vi "Arduino Stepper Motor v1.vi"() -> ()   [LabVIEW 2019, in "LabVIEW Interface for Arduino.lvlib"]
doc: "This example shows how to use the Arduino Stepper Motor API. The fritzing diagram shows use with the EasyStepper 4.3 or 4.4 motor controller."
uses:
  <vilib>/LabVIEW Interface for Arduino/LabVIEW Interface for Arduino.lvlib
  <vilib>/LabVIEW Interface for Arduino/Type Defs/Connection Type.ctl
  <vilib>/LabVIEW Interface for Arduino/Type Defs/Board Type.ctl
  <vilib>/LabVIEW Interface for Arduino/Type Defs/Pin Mode.ctl
panel:
  in  "Motor Enable/Disable":bool
  in  "Stop":bool
  in  "Stepper #":u8=1
  in  "OK Button":bool
  in  "Set Acceleration (0 to disable)":i16
  in  "# of Steps to Move":i16
  in  "Set Speed (Steps per Second)":i16=100
  out "Steps Remaining?":bool
  in  "Dial":i16(knob) scale=0.0..200.0
  in  "error in":errorcluster
  # "Preset Movement"
  # "Interactive Movement"
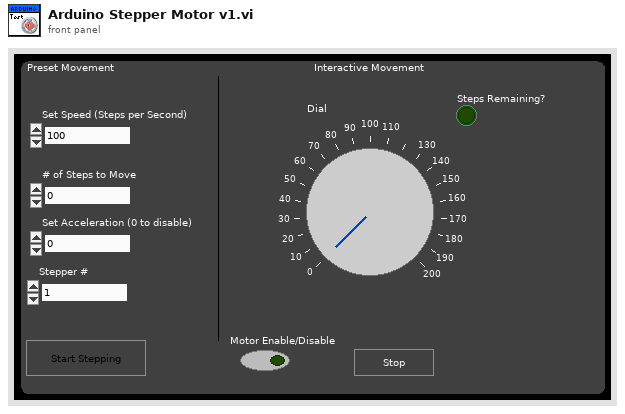
[diagram p1: front panel]
types:
  T1 = typedef "LabVIEW Interface for Arduino.lvlib/Board Type.ctl" = enum16{"Uno", "Dimuelanove w/Atmega 328", "Mega 2560"}
  T2 = typedef "LabVIEW Interface for Arduino.lvlib/Connection Type.ctl" = enum8{"USB / Serial", "XBEE", "BlueSmirf (Bluetooth)"}
  T3 = typedef "LabVIEW Interface for Arduino.lvlib/Arduino Resource.ctl" = cluster{"VISA resource":refnum<visa-resource-name>, "Board Type":T1, "Connection Type":enum8{"USB / Serial"}, "Bytes Per Packet (15)":u8}
  T4 = typedef "LabVIEW Interface for Arduino.lvlib/Pin Mode.ctl" = enum8{"Input", "Output"}
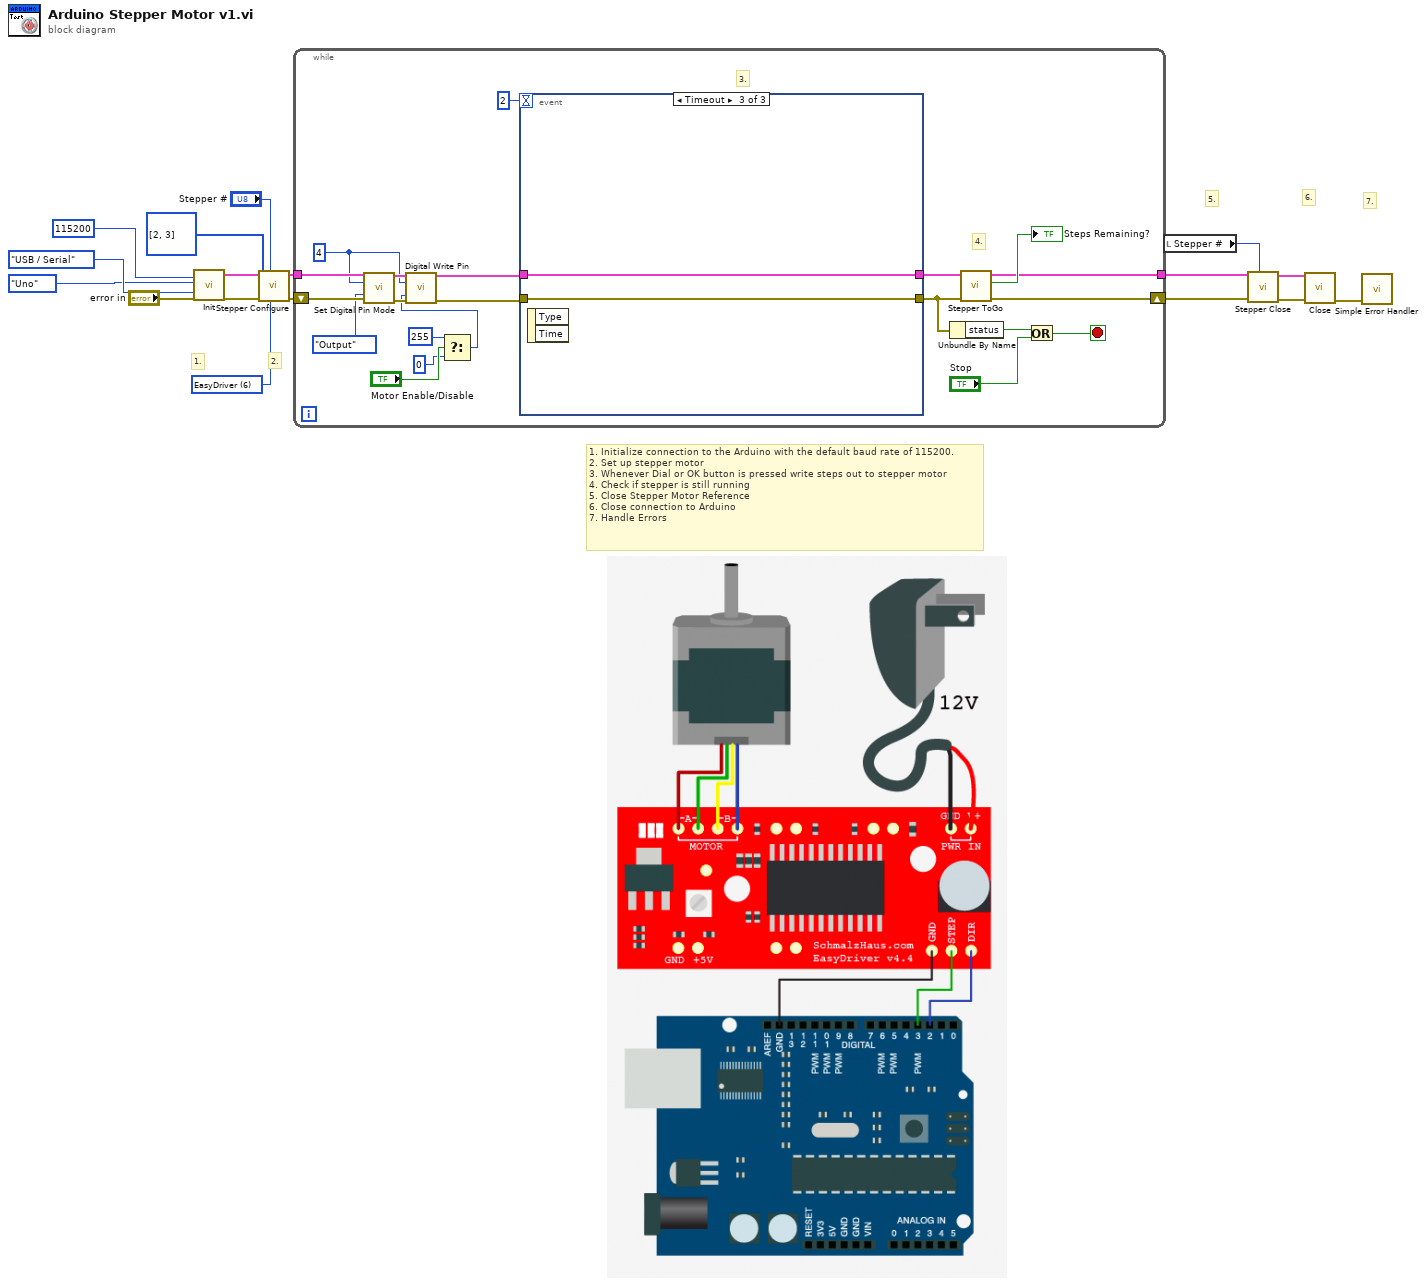
[diagram p0: block diagram]
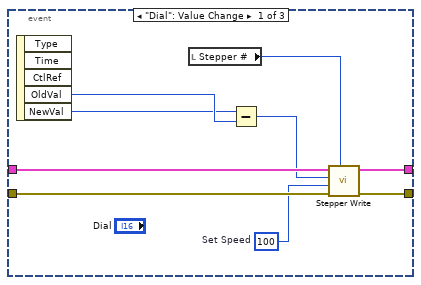
[diagram p2: hidden frame]
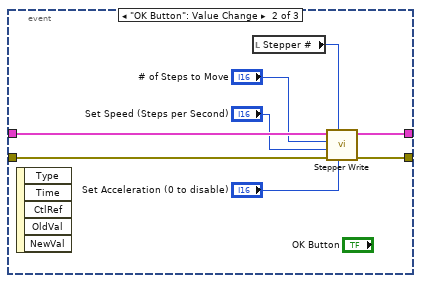
[diagram p3: hidden frame]
diagram:
  w4 = u8 6 items=["2 Wire (Pulse & Direction)"=1, "2 Wire"=2, "4 Wire"=4, "EasyDriver"=6, "AF Motor Shield (Stepper 1 & 2 Only)"=5] ("Control Method")
  # "7."
  # "6."
  # "5."
  # "2."
  # "1."
  # "1. Initialize connection to the Arduino with the default baud rate of 115200.\n2. Set up stepper motor\n3. Whenever Dial or OK button is pressed write steps out to stepper motor\n4. Check if stepper is still running\n5. Close Stepper Motor Reference \n6. Close connection to Arduino\n7. Handle Errors"
  n1 = call <vilib>:"Init.vi"("Baud Rate (115200)"=u32 115200, "Board Type (Uno)"=Board_Type."Uno", "Connection Type (USB/Serial)"=Connection_Type."USB / Serial", "error in"="error in") -> ("Arduino Resource"=w7:T3, "error out"=w6:errorcluster)  [unwired: 14 in]
  n2 = call <vilib>:"Stepper Configure.vi"("Control Method"=w4, "Stepper #"="Stepper #", "error in"=w6, "Stepper Pins"=u8[] [2, 3], "Arduino Resource"=w7) -> ("error out"=w15:errorcluster, "Arduino Resource Out"=w16:T3)  [unwired: 5 in]
  n3 = while {
    tunnel: w16 -> [w29]
    tunnel: [w33] -> w14
    shift-right: [w31] -> w13
    shift-left: w15 -> [w28]
    stop <- w37 stop-if-true
    w22 = u8 4 ("Digital I/O Pin")
    # "4."
    # "3."
    n4 = call <vilib>:"Set Digital Pin Mode.vi"("Arduino Resource"=w29, "Digital I/O Pin"=w22, "Pin Mode (Input)"=Pin_Mode."Output", "error in"=w28) -> ("Arduino Resource"=w26:T3, "error out"=w27:errorcluster)  [unwired: 10 in]
    n5 = Select(t=i16 255 ("upper limit"), s="Motor Enable/Disable", f=i16 0 ("lower limit")) -> (s? t:f=w18:i16)
    n6 = call <vilib>:"Digital Write Pin.vi"("Arduino Resource"=w26, "Digital I/O Pin (0)"=w22, "Value (0)"=w18, "error in"=w27) -> ("Arduino Resource"=w25:T3, "error out"=w24:errorcluster)  [unwired: 10 in]
    n7 = event shown="[2] Timeout" {
      selector: _ -> [_ _ _]
      dyn-events: _ -> [_ _ _]
      timeout: 2 -> [_ _ _]
      tunnel: w24 -> [w47 w54 w56]
      tunnel: w25 -> [w46 w52 w57]
      tunnel: [w45 w53 w57] -> w35
      tunnel: [w44 w55 w56] -> w32
      event "Dial": Value Change {
        w41 = i16 100  # Set Speed
        n8 = event-data() -> ("OldVal"=w43:i16, "NewVal"=w42:i16)  [unwired: 1 in, 3 out]
        n9 = local read "Stepper #"() -> (w39:u8)
        n10 = Subtract(x=w42, y=w43) -> (x-y=w40:i16)
        n11 = call <vilib>:"Stepper Write.vi"("Stepper #"=w39, "error in"=w47, "Set Speed (Steps per Second)"=w41, "# of Steps to Move"=w40, "Arduino Resource"=w46) -> ("error out"=w44:errorcluster, "Arduino Resource Out"=w45:T3)  [unwired: 5 in]
      }
      event "OK Button": Value Change {
        n12 = event-data() -> ()  [unwired: 1 in, 5 out]
        n13 = local read "Stepper #"() -> (w48:u8)
        n14 = call <vilib>:"Stepper Write.vi"("Set Acceleration (0 to disable)"="Set Acceleration (0 to disable)", "Stepper #"=w48, "error in"=w54, "Set Speed (Steps per Second)"="Set Speed (Steps per Second)", "# of Steps to Move"="# of Steps to Move", "Arduino Resource"=w52) -> ("error out"=w55:errorcluster, "Arduino Resource Out"=w53:T3)  [unwired: 4 in]
      }
      event Timeout {
        n15 = event-data() -> ()  [unwired: 1 in, 2 out]
      }
    }
    n16 = Unbundle By Name(w32) -> ("status"=w36:bool)
    n17 = call <vilib>:"Stepper ToGo.vi"("error in"=w32, "Arduino Resource"=w35) -> ("error out"=w31:errorcluster, "Steps Remaining?"=→"Steps Remaining?":bool, "Arduino Resource Out"=w33:T3)  [unwired: 6 in, 1 out]
    n18 = Or(x=w36, y="Stop") -> (x .or. y?=w37:bool)
  }
  n19 = local read "Stepper #"() -> (w8:u8)
  n20 = call <vilib>:"Stepper Close.vi"("Stepper #"=w8, "error in"=w13, "Arduino Resource"=w14) -> ("error out"=w12:errorcluster, "Arduino Resource Out"=w11:T3)  [unwired: 7 in]
  n21 = call <vilib>:"Close.vi"("Arduino Resource"=w11, "error in"=w12) -> ("error out"=w17:errorcluster)  [unwired: 13 in]
  n22 = call <vilib>:"Simple Error Handler.vi"("error in (no error)"=w17) -> ()  [unwired: 4 in, 5 out]
